vi "Config.vi"() -> ()   [LabVIEW 2020]
uses:
  Global_Variable/Global.vi
  Global_Variable/A180648.vi
  <vilib>/Utility/config.llb/NI_LVConfig.lvlib
  Libraries/S7/S7.lvlib
panel:
  in  "试验项目":cluster{"拉轴":bool, "卡簧":bool}
  in  "产品型号":string(combo)
  in  "删除":bool
  in  "确定":bool
  in  "添加":bool
  in  "退出":bool
  in  "更新":bool
  in  "选项卡控件":enum32{"产品参数"}(tab)
  in  "结果判定参数":string[][](table)=[["mm"], ["KN"], ["KN"], ["KN"], [""], [""], [""], [""], [""], [""], [""], [""]]
  in  "判定框参数":string[][](table)=[["mm"], ["KN"], ["mm"], ["KN"]]
  in  "坐标轴参数":string[][](table)=[[""], ["°/S"], ["°"], ["Nm"]]
  # "上管柱上转向轴合成"
types:
  T1 = typedef "NI_LVConfig.lvlib/Config Data RefNum.ctl" = refnum<k1>
  T2 = cluster{"[0]":cluster{string, dbl, dbl}, "[1]":cluster{string, dbl, dbl}}
  T3 = cluster{"位移":cluster{"单位":string, "下限":dbl, "上限":dbl}, "压力":cluster{"单位":string, "下限":dbl, "上限":dbl}}
  T4 = cluster{"[0]":cluster{string, dbl, dbl}, "[1]":cluster{string, dbl, dbl}, "[2]":cluster{string, dbl, dbl}, "[3]":cluster{string, dbl, dbl}}
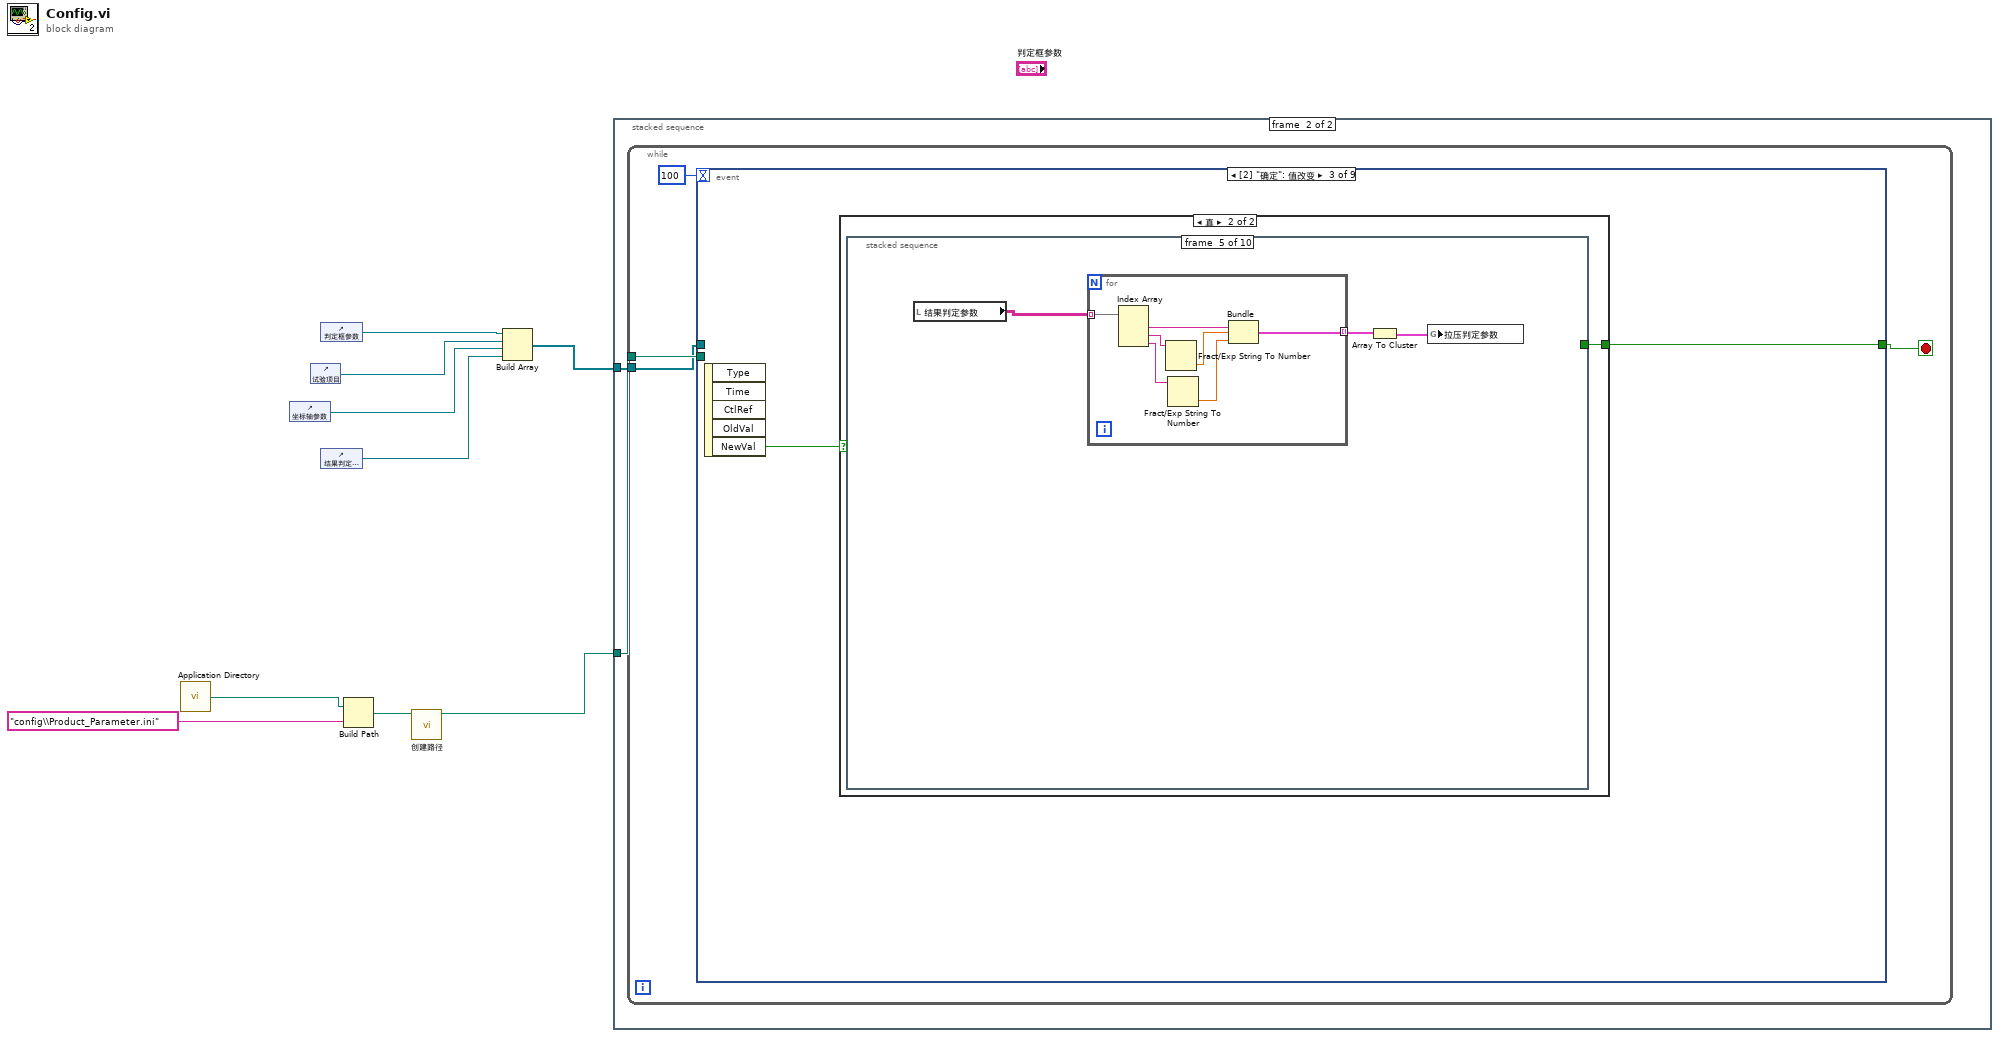
[diagram p0: block diagram]
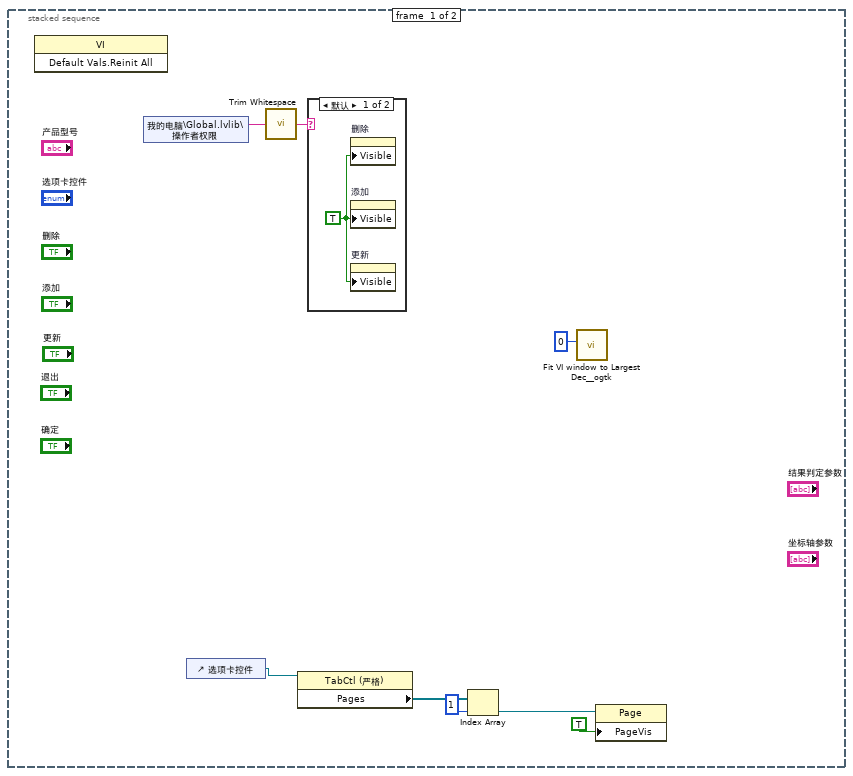
[diagram p2: hidden frame]
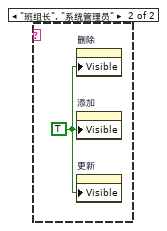
[diagram p3: hidden frame]
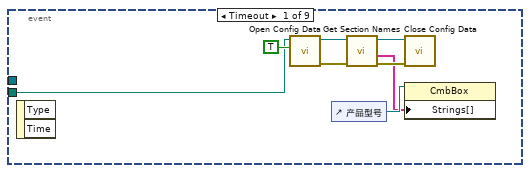
[diagram p4: hidden frame]
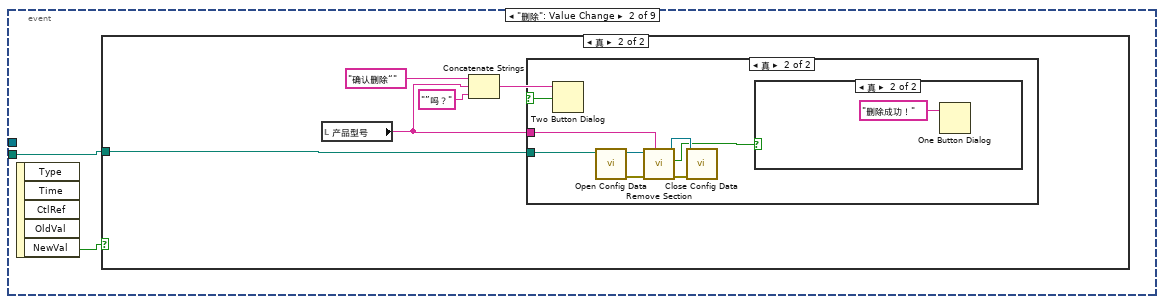
[diagram p5: hidden frame]
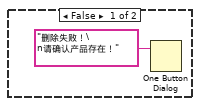
[diagram p8: hidden frame]
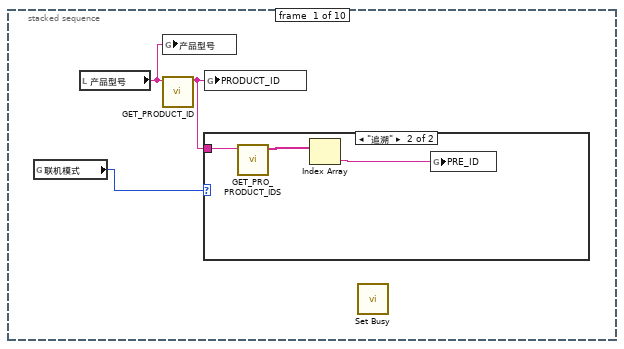
[diagram p10: hidden frame]
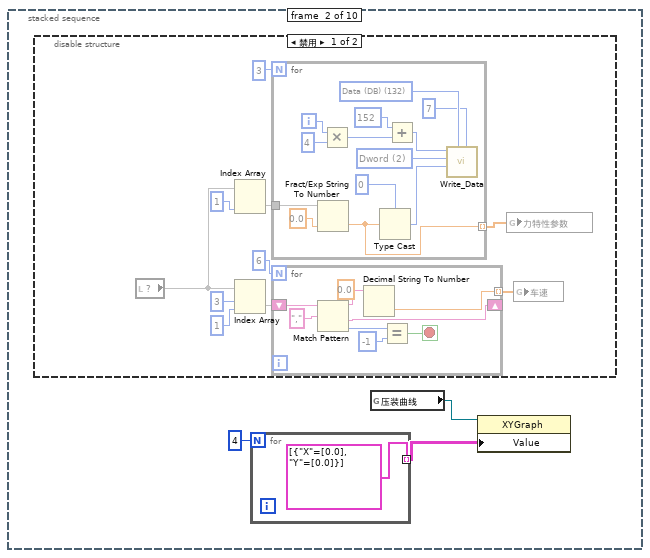
[diagram p12: hidden frame]
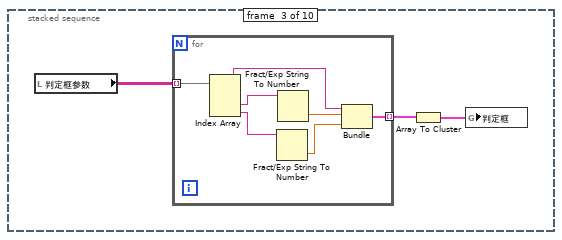
[diagram p14: hidden frame]
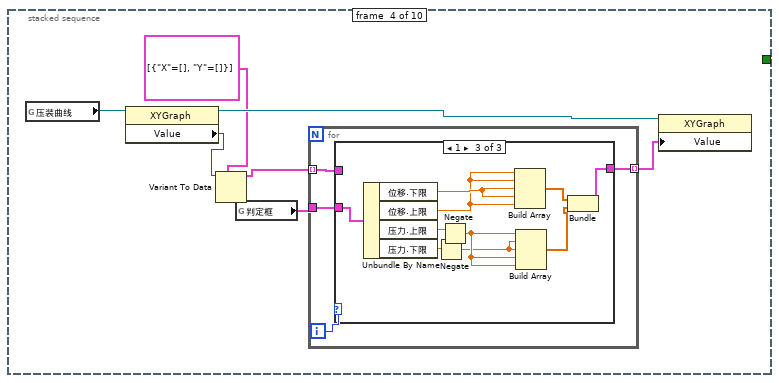
[diagram p15: hidden frame]
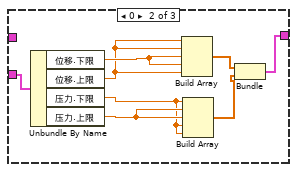
[diagram p17: hidden frame]
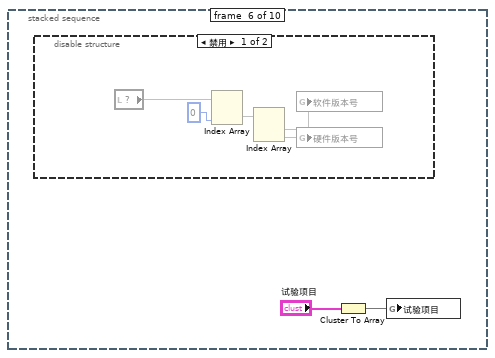
[diagram p18: hidden frame]
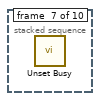
[diagram p20: hidden frame]
diagram:
  n1 = call <vilib>:"Application Directory.vi"() -> ("Application Directory"=w8:path)
  n2 = control-ref of="坐标轴参数"() -> (w3:refnum<vi>)
  n3 = control-ref of="试验项目"() -> (w4:refnum<vi>)
  n4 = control-ref of="判定框参数"() -> (w1:refnum<vi>)
  n5 = control-ref of="结果判定参数"() -> (w2:refnum<vi>)
  n6 = Build Path(base path=w8, name or relative path="config\\Product_Parameter.ini" ("名称或相对路径")) -> (appended path=w6:path)
  n7 = call "创建路径.vi"("path"=w6) -> ("path out"=w5:path)  [unwired: 9 in, 1 out]
  n8 = Build Array(w1, w4, w3, w2) -> (w9:refnum<vi>[])
  n9 = stacked-sequence {
    tunnel: w9 -> [_ w21]
    tunnel: w5 -> [_ w20]
    frame #0 {
      n10 = invoke class="VI" method="Default Vals.Reinit All"() -> ()  [unwired: 3 in, 3 out]
      n11 = shared-variable "我的电脑\\Global.lvlib\\操作者权限"() -> (w17:string)  [unwired: 1 in, 1 out]
      n12 = control-ref of="选项卡控件"() -> (w14:refnum<vi>)
      n13 = call <vilib>:"Trim Whitespace.vi"("string"=w17) -> ("trimmed string"=w16:string)  [unwired: 1 in]
      n14 = property class="TabCtl (严格)"(reference=w14) -> ("Pages"=w13:refnum<vi>[])  [unwired: 1 in, 2 out]
      n15 = case shown="默认" w16 {
        frame Default {
          w18 = TRUE ("可见")
          n16 = property on="删除" class="Bool (严格)"("Visible"=w18) -> ()  [unwired: 2 in, 2 out]
          n17 = property on="添加" class="Bool (严格)"("Visible"=w18) -> ()  [unwired: 2 in, 2 out]
          n18 = property on="更新" class="Bool (严格)"("Visible"=w18) -> ()  [unwired: 2 in, 2 out]
        }
        frame "班组长", "系统管理员" {
          w19 = TRUE ("可见")
          n19 = property on="删除" class="Bool (严格)"("Visible"=w19) -> ()  [unwired: 2 in, 2 out]
          n20 = property on="添加" class="Bool (严格)"("Visible"=w19) -> ()  [unwired: 2 in, 2 out]
          n21 = property on="更新" class="Bool (严格)"("Visible"=w19) -> ()  [unwired: 2 in, 2 out]
        }
      }
      n22 = Index Array(array=w13, index=1 ("索引")) -> (element=w12:refnum<vi>)
      n23 = call <userlib>:"Fit VI window to Largest Dec__ogtk.vi"("border spacing (2 px)"=0) -> ()  [unwired: 5 in, 2 out]
      n24 = property class="Page"(reference=w12, "PageVis"=TRUE ("选项卡可见")) -> ()  [unwired: 1 in, 2 out]
    }
    frame #1 {
      n25 = while {
        tunnel: w20 -> [w25]
        tunnel: w21 -> [w23]
        stop <- w24 stop-if-true
        n26 = event shown="[2] \"确定\": 值改变" {
          selector: _ -> [_ _ _ _ _ _ _ _ _]
          dyn-events: _ -> [_ _ _ _ _ _ _ _ _]
          timeout: 100 -> [_ _ _ _ _ _ _ _ _]
          tunnel: w25 -> [w28 w35 _ _ w162 w189 _ w213 _]
          tunnel: [_ _ w51 _ _ _ TRUE _ TRUE] -> w24
          tunnel: w23 -> [_ _ _ _ w163 w190 _ w212 _]
          event Timeout {
            n27 = event-data() -> ()  [unwired: 1 in, 2 out]
            n28 = call <vilib>:"Open Config Data.vi"("create file if necessary (T)"=TRUE, "configuration file path"=w28) -> ("error out"=w30:errorcluster, "refnum"=w29:T1)  [unwired: 7 in, 1 out]
            n29 = control-ref of="产品型号"() -> (w27:refnum<vi>)
            n30 = call <vilib>:"Get Section Names.vi"("error in (no error)"=w30, "refnum"=w29) -> ("error out"=w32:errorcluster, "section names"=w26:string[], "refnum out"=w31:T1)  [unwired: 7 in]
            n31 = call <vilib>:"Close Config Data.vi"("error in (no error)"=w32, "refnum"=w31) -> ()  [unwired: 8 in, 2 out]
            n32 = property on="属性节点" class="CmbBox"(reference=w27, "Strings[]"=w26) -> ()  [unwired: 1 in, 2 out]
          }
          event "删除": Value Change {
            n33 = event-data() -> ("NewVal"=w34:bool)  [unwired: 1 in, 4 out]
            n34 = case shown="真" w34 {
              tunnel: w35 -> [_ w37]
              frame False {
              }
              frame True {
                n35 = local read "产品型号"() -> (w36:string)
                n36 = Concatenate Strings("确认删除“", w36, "”吗？") -> (w39:string)
                n37 = Two Button Dialog(message=w39) -> (T button?=w38:bool)  [unwired: 2 in]
                n38 = case shown="真" w38 {
                  tunnel: w37 -> [_ w43]
                  tunnel: w36 -> [_ w42]
                  frame False {
                  }
                  frame True {
                    n39 = call <vilib>:"Open Config Data.vi"("configuration file path"=w43) -> ("error out"=w45:errorcluster, "refnum"=w48:T1)  [unwired: 8 in, 1 out]
                    n40 = call <vilib>:"Remove Section.vi"("section"=w42, "error in (no error)"=w45, "refnum"=w48) -> ("error out"=w47:errorcluster, "section exists?"=w44:bool, "refnum out"=w46:T1)  [unwired: 6 in]
                    n41 = call <vilib>:"Close Config Data.vi"("error in (no error)"=w47, "refnum"=w46) -> ()  [unwired: 8 in, 2 out]
                    n42 = case shown="真" w44 {
                      frame False {
                        n43 = One Button Dialog(message="删除失败！\n请确认产品存在！" ("消息")) -> ()  [unwired: 1 in, 1 out]
                      }
                      frame True {
                        n44 = One Button Dialog(message="删除成功！" ("消息")) -> ()  [unwired: 1 in, 1 out]
                      }
                    }
                  }
                }
              }
            }
          }
          event "确定": Value Change {
            n45 = event-data() -> ("NewVal"=w52:bool)  [unwired: 1 in, 4 out]
            n46 = case shown="真" w52 {
              tunnel: [_ w53] -> w51
              frame False {
              }
              frame True {
                n47 = stacked-sequence {
                  tunnel: [_ _ _ _ _ _ _ _ _ TRUE] -> w53
                  frame #0 {
                    n48 = global read "Global.vi" "联机模式"() -> (w54:enum16{"单机", "追溯"})
                    n49 = local read "产品型号"() -> (w56:string)
                    n50 = global write "Global.vi" "产品型号"(w56) -> ()
                    n51 = call "GET_PRODUCT_ID.vi"("PRODFUCT_NAME"=w56) -> ("PRODUCT_ID"=w55:string)  [unwired: 10 in]
                    n52 = case shown="\"追溯\"" w54 {
                      tunnel: w55 -> [_ w59]
                      frame "单机", Default {
                      }
                      frame "追溯" {
                        n53 = call "GET_PRO_PRODUCT_IDS.vi"("PRODUCT_ID"=w59) -> ("前序工位"=w58:string[])  [unwired: 10 in]
                        n54 = Index Array(array=w58) -> (element=w57:string)  [unwired: 1 in]
                        n55 = global write "追溯Global.vi" "PRE_ID"(w57) -> ()
                      }
                    }
                    n56 = global write "追溯Global.vi" "PRODUCT_ID"(w55) -> ()
                    n57 = call <vilib>:"Set Busy.vi"() -> ()  [unwired: 10 in, 2 out]
                  }
                  frame #1 {
                    n58 = disable-structure shown="禁用" {
                      frame Disabled {
                        n59 = local read item#-1() -> (w70)
                        n60 = Index Array(array=w70, index (col)=1 ("禁用的索引 (列)")) -> (element=w73)  [unwired: 1 in]
                        n61 = Index Array(array=w70, index (row)=3 ("索引 (行)"), index (col)=1 ("禁用的索引 (列)")) -> (element=w67)
                        n62 = for {
                          N: 3 -> [_]
                          tunnel: w73 -> [w91]
                          tunnel: [w83] -> w64 mode=indexing
                          i -> [w86]
                          w93 = u16 2 items=["byte", "word", "Dword"] ("数据类型")
                          w95 = u8 132 items=["I/O (P)"=128, "Input (I)"=129, "Output (Q)"=130, "Bit Memory (M)"=131, "Data (DB)"=132, "Instance Data (DI)"=133, "Local Data (L)"=134, "Predecessor Local Data (VL)"=135] ("寄存器类型")
                          n63 = Fract/Exp String To Number(string=w91, default (0 dbl)=sgl 0.0) -> (number=w83:sgl)  [unwired: 2 in, 1 out]
                          n64 = Multiply(x=w86, y=4) -> (x*y=w87:i32)
                          n65 = Type Cast(type=u32 0 ("写入地址"), x=w83) -> (*(type *) &x=w89:u32)
                          n66 = Add(x=u32 152 ("写入地址"), y=w87) -> (x+y=w84:u32)
                          n67 = call "Write_Data.vi"("DB #"=u16 7, "寄存器类型"=w95, "写入数据"=w89, "数据类型"=w93, "写入地址"=w84) -> ()  [unwired: 4 in, 3 out]
                        }
                        n68 = for {
                          N: 6 -> [_]
                          shift-right: [w80] -> _
                          shift-left: w67 -> [w82]
                          tunnel: [w76] -> w66 mode=indexing
                          stop <- w75 stop-if-true
                          n69 = Match Pattern(string=w82, regular expression="," ("正则表达式")) -> (before substring=w77:string, after substring=w80:string, offset past match=w79:i32)  [unwired: 1 in, 1 out]
                          n70 = Decimal String To Number(string=w77, default (0L)=sgl 0.0 ("默认(0 I32)")) -> (number=w76:sgl)  [unwired: 1 in, 1 out]
                          n71 = Equal?(x=w79, y=-1) -> (x = y?=w75:bool)
                        }
                        n72 = global write "A180648.vi" "力特性参数"(w64) -> ()
                        n73 = global write "A180648.vi" "车速"(w66) -> ()
                      }
                      frame Enabled {
                      }
                    }
                    n74 = for {
                      N: 4 -> [_]
                      tunnel: [cluster{"X":dbl[], "Y":dbl[]}[] [{"X"=[0.0], "Y"=[0.0]}]] -> w62 mode=indexing
                    }
                    n75 = global read "A180648.vi" "压装曲线"() -> (w60:refnum<vi>)
                    n76 = property class="XYGraph"(reference=w60, "Value"=w62) -> ()  [unwired: 1 in, 2 out]
                  }
                  frame #2 {
                    n77 = local read "判定框参数"() -> (w98:string[][])
                    n78 = for {
                      tunnel: w98 -> [w105] mode=indexing
                      tunnel: [w99] -> w97 mode=indexing
                      n79 = Index Array(array=w105) -> (element #1=w102:string, element #2=w104:string, element #3=w103:string)  [unwired: 3 in]
                      n80 = Fract/Exp String To Number(string=w103) -> (number=w100:dbl)  [unwired: 3 in, 1 out]
                      n81 = Fract/Exp String To Number(string=w104) -> (number=w101:dbl)  [unwired: 3 in, 1 out]
                      n82 = Bundle(w102, w101, w100) -> (w99:cluster{string, dbl, dbl})  [unwired: 1 in]
                    }
                    n83 = Array To Cluster(array=w97) -> (cluster=w96:T2)
                    n84 = global write "判定参数.vi" "判定框"(w96) -> ()
                  }
                  frame #3 {
                    n85 = global read "A180648.vi" "压装曲线"() -> (w112:refnum<vi>)
                    n86 = property class="XYGraph"(reference=w112) -> (reference out=w109:refnum<vi>, "Value"=w111:variant)  [unwired: 1 in, 1 out]
                    n87 = Variant To Data(type=cluster{"X":dbl[], "Y":dbl[]}[] [{"X"=[], "Y"=[]}], Variant=w111) -> (data=w110:cluster{"X":dbl[], "Y":dbl[]}[])  [unwired: 1 in, 1 out]
                    n88 = global read "判定参数.vi" "判定框"() -> (w106:T3)
                    n89 = for {
                      tunnel: w110 -> [w115] mode=indexing
                      tunnel: [w114] -> w107 mode=indexing
                      tunnel: w106 -> [w113]
                      i -> [w116]
                      n90 = case shown="1" w116 {
                        tunnel: w115 -> [w117 _ _]
                        tunnel: [w117 w120 w130] -> w114
                        tunnel: w113 -> [_ w125 w131]
                        frame Default {
                        }
                        frame 0 {
                          n91 = Unbundle By Name(w125) -> ("位移.下限"=w124:dbl, "位移.上限"=w123:dbl, "压力.下限"=w118:dbl, "压力.上限"=w119:dbl)
                          n92 = Build Array(w123, w123, w124, w124, w123) -> (w122:dbl[])
                          n93 = Build Array(w118, w119, w119, w118, w118) -> (w121:dbl[])
                          n94 = Bundle(w122, w121) -> (w120:cluster{dbl[], dbl[]})  [unwired: 1 in]
                        }
                        frame 1 {
                          n95 = Unbundle By Name(w131) -> ("位移.下限"=w135:dbl, "位移.上限"=w134:dbl, "压力.上限"=w128:dbl, "压力.下限"=w129:dbl)
                          n96 = Negate(x=w129) -> (-x=w126:dbl)
                          n97 = Negate(x=w128) -> (-x=w127:dbl)
                          n98 = Build Array(w134, w134, w135, w135, w134) -> (w133:dbl[])
                          n99 = Build Array(w127, w126, w126, w127, w127) -> (w132:dbl[])
                          n100 = Bundle(w133, w132) -> (w130:cluster{dbl[], dbl[]})  [unwired: 1 in]
                        }
                      }
                    }
                    n101 = property class="XYGraph"(reference=w109, "Value"=w107) -> ()  [unwired: 1 in, 2 out]
                  }
                  frame #4 {
                    n102 = local read "结果判定参数"() -> (w138:string[][])
                    n103 = for {
                      tunnel: w138 -> [w140] mode=indexing
                      tunnel: [w139] -> w136 mode=indexing
                      n104 = Index Array(array=w140) -> (element #1=w145:string, element #2=w144:string, element #3=w142:string)  [unwired: 3 in]
                      n105 = Fract/Exp String To Number(string=w144) -> (number=w143:dbl)  [unwired: 3 in, 1 out]
                      n106 = Fract/Exp String To Number(string=w142) -> (number=w141:dbl)  [unwired: 3 in, 1 out]
                      n107 = Bundle(w145, w143, w141) -> (w139:cluster{string, dbl, dbl})  [unwired: 1 in]
                    }
                    n108 = Array To Cluster(array=w136) -> (cluster=w137:T4)
                    n109 = global write "判定参数.vi" "拉压判定参数"(w137) -> ()
                  }
                  frame #5 {
                    n110 = disable-structure shown="禁用" {
                      frame Disabled {
                        n111 = local read item#-1() -> (w152)
                        n112 = Index Array(array=w152, index (col)=0 ("禁用的索引 (列)")) -> (element=w150)  [unwired: 1 in]
                        n113 = Index Array(array=w150) -> (element #1=w149, element #2=w148)  [unwired: 2 in]
                        n114 = global write "Global.vi" "软件版本号"(w149) -> ()
                        n115 = global write "Global.vi" "硬件版本号"(w148) -> ()
                      }
                      frame Enabled {
                      }
                    }
                    n116 = Cluster To Array(cluster="试验项目") -> (array=w147:bool[])
                    n117 = global write "Global.vi" "试验项目"(w147) -> ()
                  }
                  frame #6 {
                    n118 = call <vilib>:"Unset Busy.vi"() -> ()  [unwired: 11 in, 1 out]
                  }
                  frame #7 {
                    n119 = global read "Global.vi" "更换产品"() -> (w154:refnum<vi>)
                    n120 = vi-ref "Auto.vi"() -> (w153:refnum<vi>)
                    n121 = property class="VIRef"(reference=w154, "Val(Sgnl)"=w153) -> ()  [unwired: 1 in, 2 out]
                  }
                  frame #8 {
                    w155 = 64 items=["None"=0, "Hand, Error, Stop"=16, "Question"=32, "Exclamation, Warning"=48, "Asterisk, Information"=64] ("icon")
                    w157 = "参数装载成功！" ("消息")
                    n122 = call "浮动通知.vi"("通知内容"=w157) -> ()  [unwired: 11 in]
                    n123 = call "信息框（标题、文本、图标）.vi"("icon"=w155, "caption"="参数加载", "text"=w157) -> ()  [unwired: 7 in, 2 out]
                  }
                  frame #9 {
                    n124 = control-ref of="本VI"() -> (w158:refnum<vi>)
                    n125 = invoke class="VI" method="FP.Close"(reference=w158) -> ()  [unwired: 2 in, 3 out]
                  }
                }
              }
            }
          }
          event "试验项目.卡簧": Value Change {
            n126 = event-data() -> ("NewVal"=w160:bool)  [unwired: 1 in, 5 out]
            n127 = case shown="真" w160 {
              frame False {
              }
              frame True {
                (unwired) FALSE ("值")
              }
            }
          }
          event "添加": Value Change {
            n128 = event-data() -> ("NewVal"=w161:bool)  [unwired: 1 in, 4 out]
            n129 = case shown="真" w161 {
              tunnel: w163 -> [_ w167]
              tunnel: w162 -> [_ w166]
              frame False {
              }
              frame True {
                n130 = call "产品添加提示：用户输入"() -> ("产品型号"=w164:string, "确定"=w165:bool)  [unwired: 17 in, 1 out]
                n131 = case shown="真" w165 {
                  tunnel: w167 -> [_ w170]
                  tunnel: w166 -> [_ w169]
                  tunnel: w164 -> [_ w168]
                  frame False {
                  }
                  frame True {
                    n132 = case shown="默认" w168 {
                      selector: w168 -> [_ w173]
                      tunnel: w170 -> [_ w176]
                      tunnel: w169 -> [_ w175]
                      frame "" {
                        n133 = One Button Dialog(message="产品名称不得为空!" ("text")) -> ()  [unwired: 1 in, 1 out]
                      }
                      frame Default {
                        n134 = property on="产品型号" class="CmbBox"() -> ("Strings[]"=w174:string[])  [unwired: 2 in, 2 out]
                        n135 = Search 1D Array(1D array=w174, element=w173) -> (index of element=w172:i32)  [unwired: 1 in]
                        n136 = case shown="-1" w172 {
                          tunnel: w176 -> [_ w180]
                          tunnel: w175 -> [_ w179]
                          tunnel: w173 -> [_ w178]
                          frame Default {
                            n137 = One Button Dialog(message="产品已存在！" ("消息")) -> ()  [unwired: 1 in, 1 out]
                          }
                          frame -1 {
                            n138 = stacked-sequence {
                              tunnel: w180 -> [w186 _]
                              tunnel: w179 -> [w185 _]
                              tunnel: w178 -> [w184 _]
                              frame #0 {
                                n139 = call <vilib>:"Set Busy.vi"() -> ("error out"=w182:errorcluster)  [unwired: 10 in, 1 out]
                                n140 = call "Read_Write INI File.vi"("Mode"=enum16{"Read", "Write"}."Write", "Section"=w184, "error in"=w182, "Filepath"=w185, "Ctl Refnum"=w186) -> ("error out"=w181:errorcluster)  [unwired: 6 in]
                                n141 = call <vilib>:"Unset Busy.vi"("error in (no error)"=w181) -> ()  [unwired: 10 in, 1 out]
                              }
                              frame #1 {
                                n142 = One Button Dialog(message="添加成功！" ("消息")) -> ()  [unwired: 1 in, 1 out]
                              }
                            }
                          }
                        }
                      }
                    }
                  }
                }
              }
            }
          }
          event "产品型号": Value Change {
            n143 = event-data() -> ("NewVal"=w188:string)  [unwired: 1 in, 4 out]
            n144 = stacked-sequence {
              tunnel: w190 -> [_ _ w194]
              tunnel: w189 -> [_ _ w193]
              tunnel: w188 -> [_ w192 _]
              frame #0 {
                n145 = control-ref of="本VI"() -> (w191:refnum<vi>)
                n146 = invoke class="VI" method="Default Vals.Reinit All"(reference=w191) -> ()  [unwired: 2 in, 3 out]
              }
              frame #1 {
                n147 = local write "产品型号"(w192) -> ()
              }
              frame #2 {
                n148 = disable-structure shown="启用" {
                  disable-tunnel: w194 -> [w196 w205]
                  disable-tunnel: w193 -> [w195 w206]
                  frame Disabled {
                    n149 = for {
                      tunnel: w196 -> [w199] mode=indexing
                      tunnel: w195 -> [w198]
                      n150 = local read "产品型号"() -> (w197:string)
                      n151 = call "Read_Write ParaINI File.vi"("Mode"=enum16{"Read", "Write"}."Read", "Section"=w197, "Filepath"=w198, "Ctl Refnum"=w199) -> ()  [unwired: 7 in, 1 out]
                    }
                  }
                  frame Enabled {
                    n152 = call <vilib>:"Set Busy.vi"() -> ("error out"=w201:errorcluster)  [unwired: 10 in, 1 out]
                    n153 = local read "产品型号"() -> (w204:string)
                    n154 = call "Read_Write INI File.vi"("Mode"=enum16{"Read", "Write"}."Read", "Section"=w204, "error in"=w201, "Filepath"=w206, "Ctl Refnum"=w205) -> ("error out"=w202:errorcluster)  [unwired: 6 in]
                    n155 = call <vilib>:"Unset Busy.vi"("error in (no error)"=w202) -> ()  [unwired: 10 in, 1 out]
                  }
                }
              }
            }
          }
          event "退出": Value Change {
            n156 = event-data() -> ()  [unwired: 1 in, 5 out]
            n157 = control-ref of="本VI"() -> (w209:refnum<vi>)
            n158 = invoke class="VI" method="FP.Close"(reference=w209) -> (reference out=w207:refnum<vi>, error out=w208:errorcluster)  [unwired: 2 in, 1 out]
            n159 = Close Reference(reference=w207, error in (no error)=w208) -> ()  [unwired: 1 out]
          }
          event "更新": Value Change {
            n160 = event-data() -> ("NewVal"=w211:bool)  [unwired: 1 in, 4 out]
            n161 = case shown="真" w211 {
              tunnel: w213 -> [_ w216]
              tunnel: w212 -> [_ w215]
              frame False {
              }
              frame True {
                n162 = disable-structure shown="启用" {
                  disable-tunnel: w216 -> [w219 w230]
                  disable-tunnel: w215 -> [w218 w225]
                  disable-tunnel: [w217 w227] -> w214
                  frame Disabled {
                    n163 = for {
                      tunnel: w219 -> [w222]
                      tunnel: w218 -> [w221] mode=indexing
                      tunnel: [w220] -> w217
                      n164 = local read "产品型号"() -> (w224:string)
                      n165 = call "Read_Write ParaINI File.vi"("Mode"=enum16{"Read", "Write"}."Write", "Section"=w224, "Filepath"=w222, "Ctl Refnum"=w221) -> ("error out"=w220:errorcluster)  [unwired: 7 in]
                    }
                  }
                  frame Enabled {
                    n166 = call <vilib>:"Set Busy.vi"() -> ("error out"=w226:errorcluster)  [unwired: 10 in, 1 out]
                    n167 = local read "产品型号"() -> (w229:string)
                    n168 = call "Read_Write INI File.vi"("Mode"=enum16{"Read", "Write"}."Write", "Section"=w229, "error in"=w226, "Filepath"=w230, "Ctl Refnum"=w225) -> ("error out"=w227:errorcluster)  [unwired: 6 in]
                  }
                }
                n169 = case shown="无错误" w214 {
                  frame No Error {
                    n170 = call <vilib>:"Unset Busy.vi"() -> ()  [unwired: 11 in, 1 out]
                    n171 = Wait (ms)(milliseconds to wait=u32 500 ("等待时间（毫秒）")) -> ()  [unwired: 1 out]
                    n172 = One Button Dialog(message="更新成功！" ("通知内容")) -> ()  [unwired: 1 in, 1 out]
                  }
                  frame Error {
                    n173 = Wait (ms)(milliseconds to wait=u32 500 ("等待时间（毫秒）")) -> ()  [unwired: 1 out]
                    n174 = call "浮动通知.vi"("通知内容"="更新失败！") -> ()  [unwired: 11 in]
                  }
                }
              }
            }
          }
          event Panel Close {
            n175 = event-data() -> ()  [unwired: 1 in, 3 out]
          }
        }
      }
    }
  }
